vi "DAQ - Get Attributes.vi"(0 "reference in":refnum<class "GSwFormDSP.lvclass">, 5 "error in (no error)":errorcluster) -> (13 "Monitoring Attributes":string[][](array[string]), 14 "reference in":refnum<class "GSwFormDSP.lvclass">, 19 "error out":errorcluster)   [LabVIEW 2020, in "GSwFormDSP.lvclass"]
uses:
  GSwFormDSP.lvclass
  functions/Attribute List.ctl
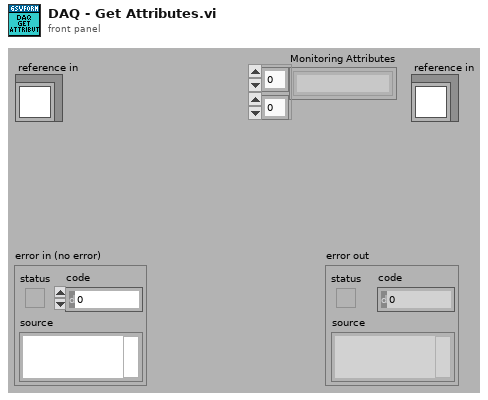
[diagram p1: front panel]
types:
  T1 = typedef "GSwFormDSP.lvclass/Attribute List.ctl" = string
  T2 = typedef "GSwFormDSP.lvclass/ObjectAttributes.ctl" = cluster{"Wform Ref":refnum<data-value>, "Nb Signals":i32, "Spectral Function Parameters":T3, "FFT":waveform(cdb)[], "Nb FFT":i32, "Nb Averages":i32[], "Reference Indexes":i32[], "Response Indexes":i32[], "Coherence":waveform(dbl)[], "TDF Parameters":T5, "DAQ":cluster{"Duration (sec)":dbl, "Buffer Size (Samples)":i32, "Offset (Samples)":i32}, "Filter Impulse Response (TDF)":waveform(dbl), "Sound Playback":T6}
  T3 = typedef "GSwFormDSP.lvclass/Spectral Parameters.ctl" = cluster{"Frequency resolution (Hz)":dbl, "Overlap":dbl, "Window":T4}
  T4 = typedef "NI_AALPro.lvlib/windowTd.ctl" = u32
  T5 = typedef "GSwFormDSP.lvclass/TDF Parameters.ctl" = cluster{"Filter":enum32{"Lowpass", "Highpass", "Bandpass", "Bandstop"}, "Type:":enum16{"Butterworth", "Chebyshev", "Inv Chebyshev", "Elliptic", "Bessel"}, "LP cutoff freq":dbl, "HP cutoff freq":dbl, "Order":i32, "passband ripple (dB)":dbl, "stopband attenuation (dB)":dbl, "Phaseless Filter":bool, "Include Fade IN and OUT":bool}
  T6 = typedef "GSwFormDSP.lvclass/Sound Playback.ctl" = cluster{"Timer start (ms)":u32, "task ID":T7, "Cursor Init Location (s)":dbl, "SC Volume":dbl}
  T7 = typedef "Sound Output Task ID.ctl" = u32
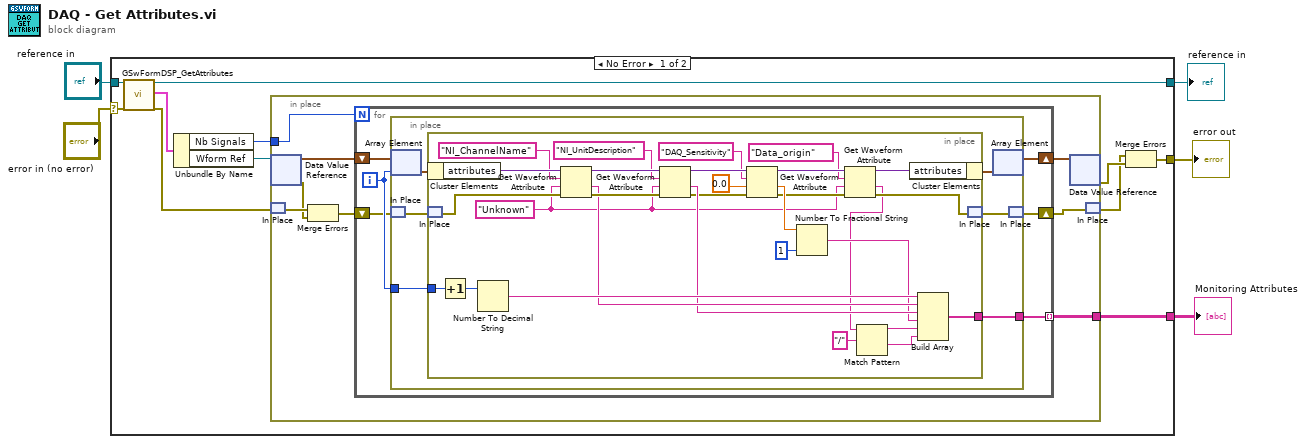
[diagram p0: block diagram]
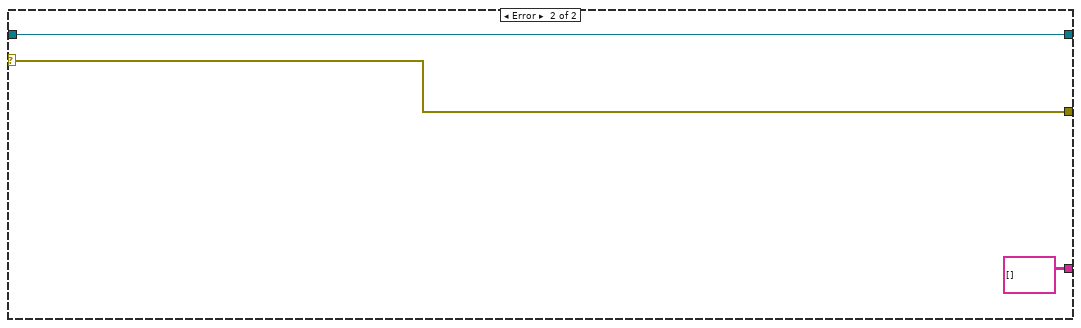
[diagram p2: hidden frame]
diagram:
  n1 = case shown="No Error" "error in (no error)" {
    selector: "error in (no error)" -> [w13 w68]
    tunnel: [w16 w68] -> w4
    tunnel: [w14 w67] -> w2
    tunnel: "reference in" -> [w15 w67]
    tunnel: [w6 string[][] []] -> w1
    frame No Error {
      n2 = call "GSwFormDSP_GetAttributes.vi"("reference in"=w15, "error in (no error)"=w13) -> ("reference out"=w14:refnum<class "GSwFormDSP.lvclass">, "attributes"=w12:T2, "error out"=w10:errorcluster)  [unwired: 14 in, 1 out]
      n3 = Unbundle By Name(w12) -> ("Nb Signals"=w9:i32, "Wform Ref"=w11:refnum<data-value>)
      n4 = in-place {
        in-place-border: w9 -> [w20]
        in-place-border: [w17] -> w6
        n5 = in-place-dvr #1(w11) -> (w24:waveform(dbl)[], w21:errorcluster)
        n6 = in-place-match #2(w10) -> (w22:errorcluster)
        n7 = Merge Errors(w22, w21) -> (w19:errorcluster)
        n8 = for {
          N: w20 -> [_]
          shift-right: [w29] -> w23
          shift-left: w24 -> [w30]
          shift-right: [w26] -> w18
          shift-left: w19 -> [w27]
          tunnel: [w25] -> w17 mode=indexing
          i -> [w28]
          n9 = in-place {
            in-place-border: w28 -> [w34]
            in-place-border: [w31] -> w25
            n10 = in-place-array #3(w30, w28) -> (w36:waveform(dbl))
            n11 = in-place-match #4(w27) -> (w33:errorcluster)
            n12 = in-place {
              in-place-border: w34 -> [w64]
              in-place-border: [w37] -> w31
              w44 = "Unknown"
              n13 = in-place-cluster #5(w36) -> ("attributes"=w60:variant)
              n14 = in-place-match #6(w33) -> (w62:errorcluster)
              n15 = Increment(x=w64) -> (x+1=w65:i32)
              n16 = Number To Decimal String(number=w65) -> (decimal integer string=w63:string)  [unwired: 1 in]
              n17 = Get Waveform Attribute(4:w62, 5:w44, 6:T1 "NI_ChannelName" ("Attribute List"), 7:w60) -> (0:w61:errorcluster, 1:w56:string, 3:w59:variant)  [unwired: 1 out]
              n18 = Get Waveform Attribute(4:w61, 5:w44, 6:T1 "NI_UnitDescription" ("Attribute List"), 7:w59) -> (0:w53:errorcluster, 1:w54:string, 3:w58:variant)  [unwired: 1 out]
              n19 = Get Waveform Attribute(4:w53, 5:0.0, 6:T1 "DAQ_Sensitivity" ("Attribute List"), 7:w58) -> (0:w46:errorcluster, 1:w50:dbl, 3:w47:variant)  [unwired: 1 out]
              n20 = Number To Fractional String(number=w50, precision (6)=i16 1) -> (F-format string=w48:string)  [unwired: 2 in]
              n21 = Get Waveform Attribute(4:w46, 5:w44, 6:T1 "Data_origin" ("Attribute List"), 7:w47) -> (0:w42:errorcluster, 1:w41:string, 3:w43:variant)  [unwired: 1 out]
              n22 = Match Pattern(string=w41, regular expression="/") -> (before substring=w39:string, after substring=w38:string)  [unwired: 1 in, 2 out]
              n23 = in-place-cluster #5("attributes"=w43) -> (w35:waveform(dbl))
              n24 = Build Array(w63, w56, w54, w48, w39, w38) -> (w37:string[])
              n25 = in-place-match #6(w42) -> (w32:errorcluster)
            }
            n26 = in-place-array #3(w35) -> (w29:waveform(dbl)[])  [unwired: 1 out]
            n27 = in-place-match #4(w32) -> (w26:errorcluster)
          }
        }
        n28 = in-place-dvr #1(w23) -> (w8:errorcluster)  [unwired: 1 out]
        n29 = in-place-match #2(w18) -> (w7:errorcluster)
      }
      n30 = Merge Errors(w7, w8) -> (w16:errorcluster)
    }
    frame Error {
    }
  }
  "error out" <- w4
  "reference in" <- w2
  "Monitoring Attributes" <- w1
